vi "O2 main.vi"() -> ()   [LabVIEW 2020, in "O2 Dichtheitstest.lvlib"]
uses:
  O2 Dichtheitstest.lvlib
  O2 Settings.ctl
  Visualisierungs Elemente/Auswahlfeld.ctl
  Aktion O2 Test.ctl
  Aktion FGV O2 Leak.ctl
  Seiten/FT-IR/FGV FT-IR Gasliste Aktionen.ctl
  Seiten/CalGas Aufschaltung/FGV CalGas Aktionen.ctl
  Sprachverwaltung/FGV Aktion Tabelle zerlegen.ctl
  Messdaten/Aktionen FGV Messdaten.ctl
  Funktionstasten/Funktionstasten-Aktion.ctl
  Funktionstasten/Zustaende.ctl
  Seiten/FT-IR/FGV FT-IR Parameter.vi
  Allgemein/allgemeine Sub-VIs.lvlib
  Seiten/FT-IR/FT-IR.lvlib
  Funktionstasten/Funktionstasten.lvlib
  Seiten/CalGas Aufschaltung/CalGas Aufschaltung.lvlib
  Messdaten/Messdaten.lvlib
  Seiten/Grafik/Grafik.lvlib
  Linearisierung V2/Protokoll/Protokoll.lvlib
  Sprachverwaltung/Sprachverwaltung.lvlib
panel:
  out "Result: O2 2":sgl caption="Ergebnis: O2" format="%#.3f"
  out "Messgasdruck":sgl format="%.3f"
  out "Bestanden MGD":bool caption="Boolesch"
  out "Bestanden O2":bool caption="Boolesch"
  out "Graph":waveform(dbl)(graph) caption="Graph1"
  out "Index":i32
  out "Result: Meassuring gas pressure":sgl caption="Ergebnis: Messgasdruck" format="%#.1f"
  out "O2":sgl format="%.3f"
  out "Zeit":sgl
  in  "Textname:":string
  in  "Pfad:":path=path "D:/IAG_Data/Log"
  in  "Speichern":bool
  out "Result: O2":sgl caption="Ergebnis: O2" format="%#.3f"
  in  "Abbrechen":bool
  in  "Test Start":bool
  out "Status":string
  in  "O2 Settings":T1 {"Grenzwert: Messgasdruck 2" format="%#.1f"; "Grenzwert: Messgasdruck" format="%#.1f"; "Grenzwert: O2" format="%#.3f"; "Datenerfassungszeit:" format="%#.1f"; "Nullgas Aufschaltzeit:" format="%#.1f"; "Aufschaltpunkt" items=["Filterblock", "Analysator direkt", "PNS", "Entnahme", "Gasdivider"]; "Kalibriergas" items=["Stickstoff"]}
  # "kPa"
  # "sec"
  # "%"
  # "%"
  # "kPa"
  # "Protokoll"
  # "Ergebnis"
  # "Test - Sequenz"
  # "sec"
  # "%"
  # "-"
  # "kPa"
  # "kPa"
  # "Einstellungen"
  # "O2 Dichtheitstest"
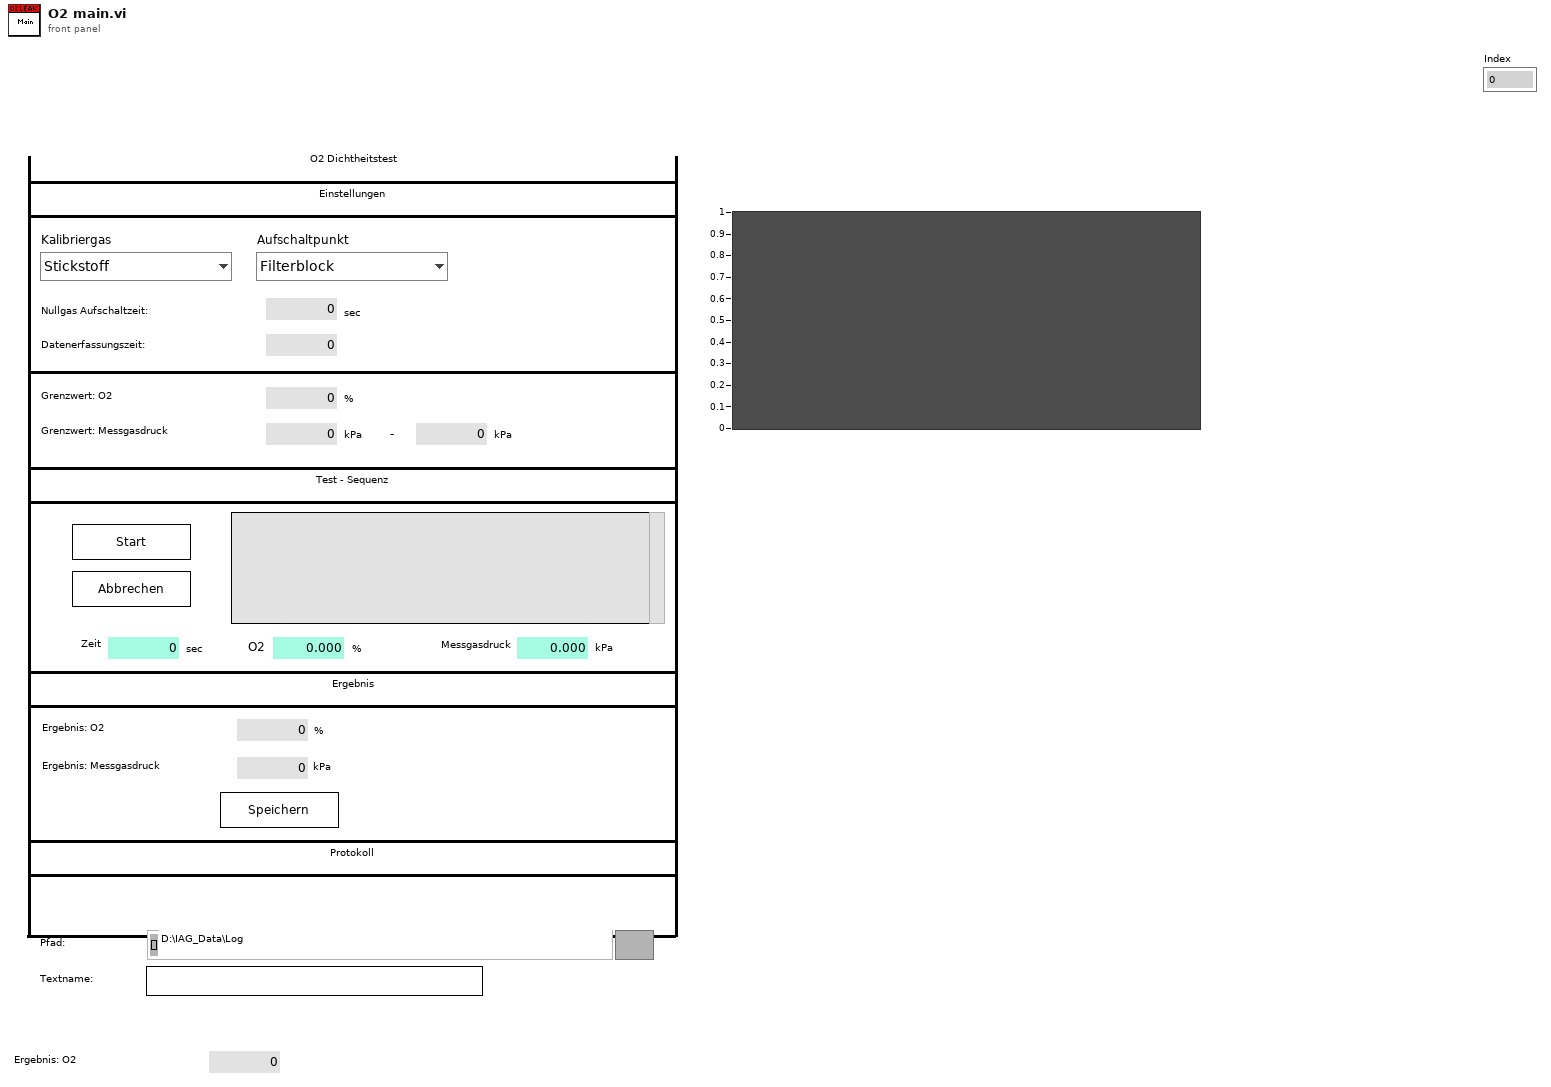
[diagram p1: front panel]
types:
  T1 = typedef "O2 Dichtheitstest.lvlib/O2 Settings.ctl" = cluster{"Kalibriergas":T2, "Aufschaltpunkt":T2, "Nullgas Aufschaltzeit:":sgl, "Datenerfassungszeit:":sgl, "Grenzwert: O2":sgl, "Grenzwert: Messgasdruck":sgl, "Grenzwert: Messgasdruck 2":sgl}
  T2 = typedef "Auswahlfeld.ctl" = u16
  T3 = typedef "O2 Dichtheitstest.lvlib/Aktion O2 Test.ctl" = enum16{"lesen", "ini", "0-Gas", "Auswerten", "Fertig"}
  T4 = typedef "Sprachverwaltung.lvlib/FGV Aktion Tabelle zerlegen.ctl" = enum16{"laden", "vereinzeln", "speichern"}
  T5 = typedef "CalGas Aufschaltung.lvlib/FGV CalGas Aktionen.ctl" = enum16{"lesen", "Analysator Auswahl", "Def.CalGas", "Aufschaltung CalGas", "laden", "speichern", "KAL extrahieren"}
  T6 = enum8{"Enabled", "Disabled", "Disabled and Grayed Out"}
  T7 = typedef "FT-IR.lvlib/FGV FT-IR Gasliste Aktionen.ctl" = enum16{"lesen", "Gasliste FT-IR", "Gasliste ausgelesen", "laden", "speichern", "löschen"}
  T8 = typedef "O2 Dichtheitstest.lvlib/Aktion FGV O2 Leak.ctl" = enum16{"lesen", "O2 settings", "Pfad", "Protokoll", "laden", "speichern"}
  T9 = typedef "String - Ausgabefeld.ctl" = string
  T10 = typedef "CalGas Aufschaltung.lvlib/Definition CalGas Anzeige.ctl" = cluster{"Namen":T11, "Werte":T13, "Werte 2":T13, "Einheit":T15, "Messbereiche":T16}
  T11 = typedef "CalGas Aufschaltung.lvlib/CalGas-Namen.ctl" = cluster{"Name":T12, "Name 2":T12, "Name 3":T12, "Name 4":T12, "Name 5":T12, "Name 6":T12, "Name 7":T12, "Name 8":T12, "Name 9":T12, "Name 10":T12, "Name 11":T12, "Name 12":T12}
  T12 = typedef "String - Eingabefeld.ctl" = string
  T13 = typedef "CalGas Aufschaltung.lvlib/CalGas-Werte.ctl" = cluster{"Konzentration 1":T14, "Konzentration 2":T14, "Konzentration 3":T14, "Konzentration 4":T14, "Konzentration 5":T14, "Konzentration 6":T14, "Konzentration 7":T14, "Konzentration 8":T14, "Konzentration 9":T14, "Konzentration 10":T14, "Konzentration 11":T14, "Konzentration 12":T14}
  T14 = typedef "Zahlen-Eingabefeld.ctl" = sgl
  T15 = typedef "CalGas Aufschaltung.lvlib/CalGas-Einheit.ctl" = cluster{"Einheit 1":T2, "Einheit 2":T2, "Einheit 3":T2, "Einheit 4":T2, "Einheit 5":T2, "Einheit 6":T2, "Einheit 7":T2, "Einheit 8":T2, "Einheit 9":T2, "Einheit 10":T2, "Einheit 11":T2, "Einheit 12":T2}
  T16 = typedef "CalGas Aufschaltung.lvlib/CalGas-Messbereiche.ctl" = cluster{"Messbereich 1":T2, "Messbereich 2":T2, "Messbereich 3":T2, "Messbereich 4":T2, "Messbereich 5":T2, "Messbereich 6":T2, "Messbereich 7":T2, "Messbereich 8":T2, "Messbereich 9":T2, "Messbereich 10":T2, "Messbereich 11":T2, "Messbereich 12":T2}
  T17 = typedef "Messdaten.lvlib/Aktionen FGV Messdaten.ctl" = enum16{"lesen", "schreiben", "löschen", "Mittelwerte", "Komponente"}
  T18 = typedef "Funktionstasten.lvlib/Zustaende.ctl" = enum16{"Standby", "Pause", "Eco", "Messen", "Kalibrieren", "Spülen Filter", "Spülen Leitung", "Umgebungsluft", "0-Gas", "Cal-Gas", "CG zu PNS", "-------------", "Init 1", "Init 2", "Init 3", "Init 4", "Messen vorbereiten", "Messen durchführen", "Exit"}
  T19 = typedef "Funktionstasten.lvlib/Funktionstasten-Aktion.ctl" = enum16{"Initialisieren", "Zustand setzen", "Taste gedrückt", "Fehler speichern", "Lesen", "Manuell", "Remote", "Bitparallel", "Samplepoint", "Zeit Prüfen", "reset Umschalten"}
  T20 = typedef "O2 Dichtheitstest.lvlib/Protokoll LeakTest.ctl" = cluster{"O2":sgl, "Messgasdruck":sgl, "Startzeit":timestamp, "Endzeit":timestamp, "Bestanden?":bool}
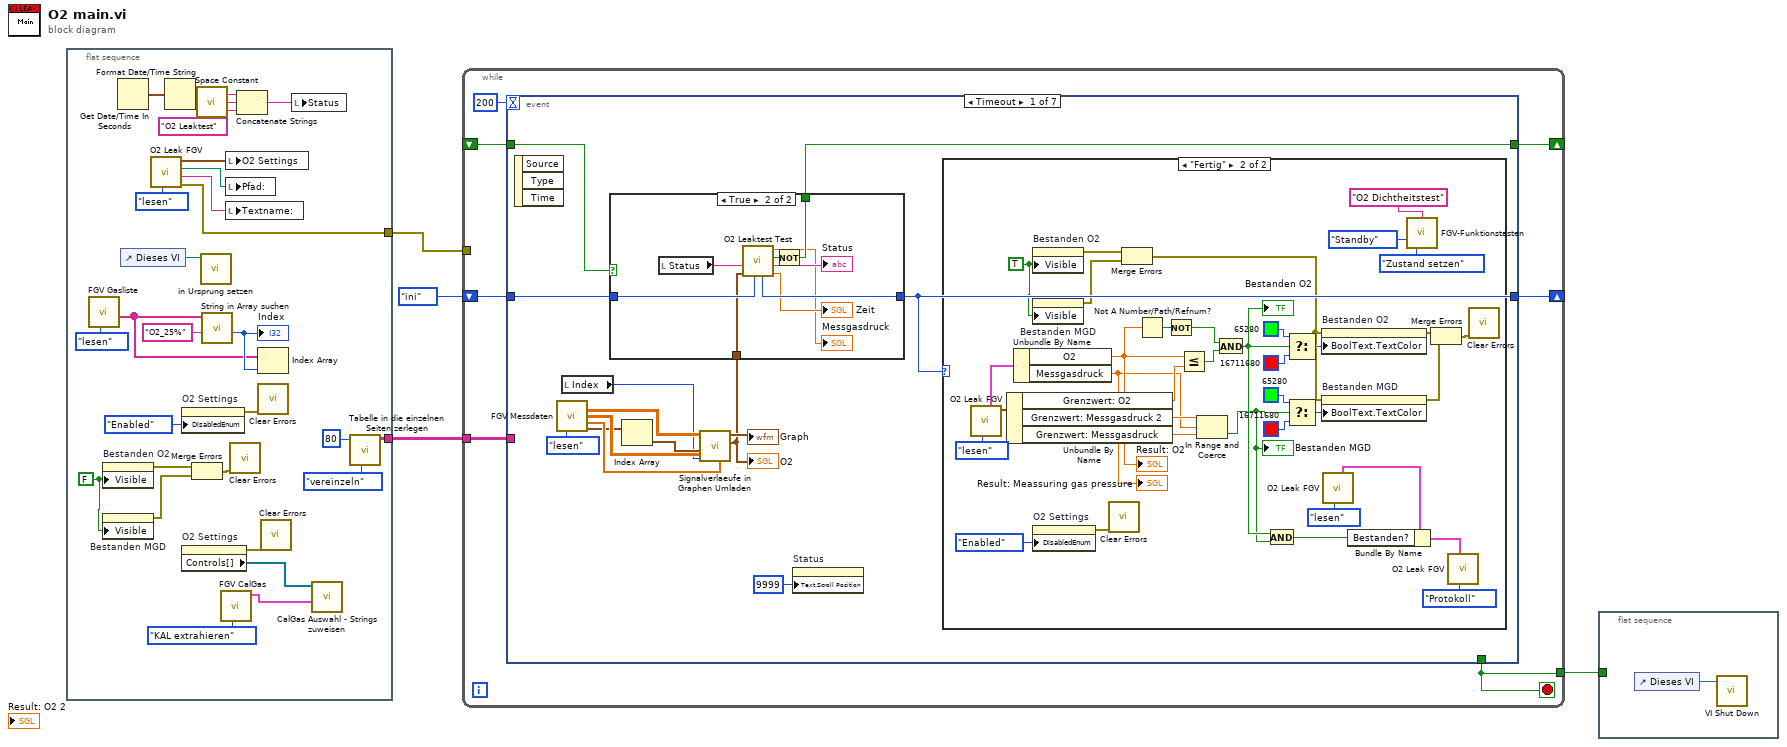
[diagram p0: block diagram]
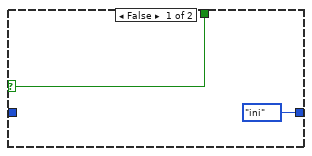
[diagram p3: hidden frame]
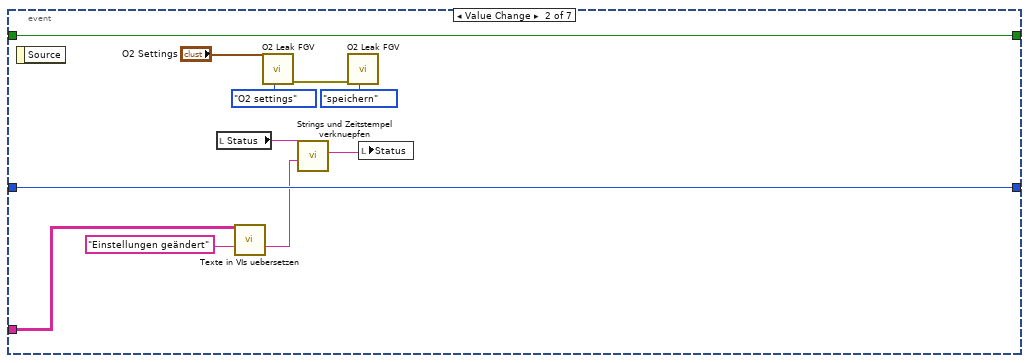
[diagram p4: hidden frame]
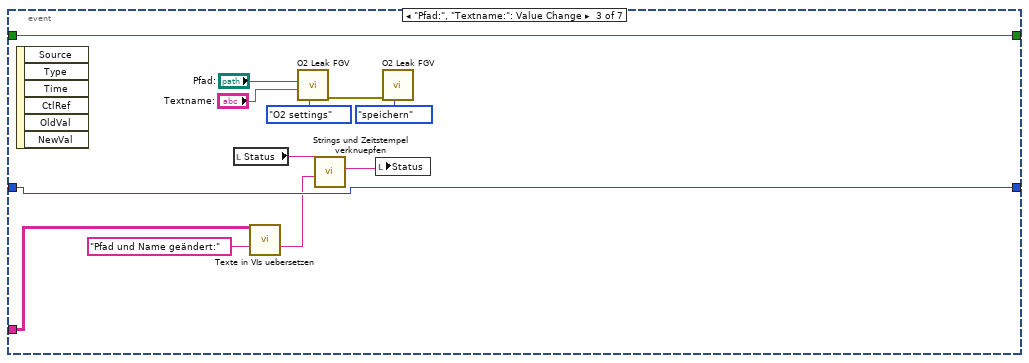
[diagram p5: hidden frame]
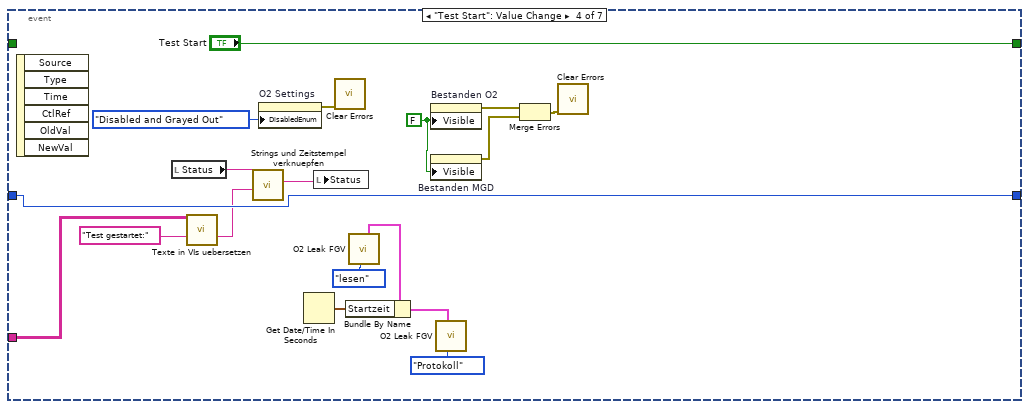
[diagram p6: hidden frame]
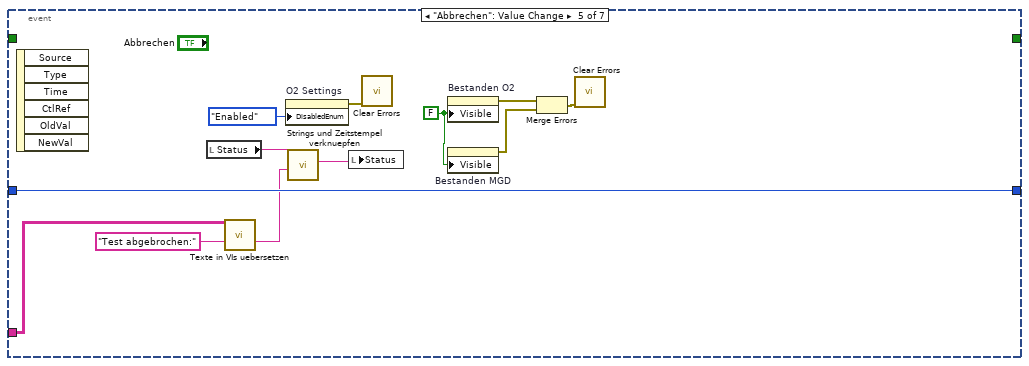
[diagram p7: hidden frame]
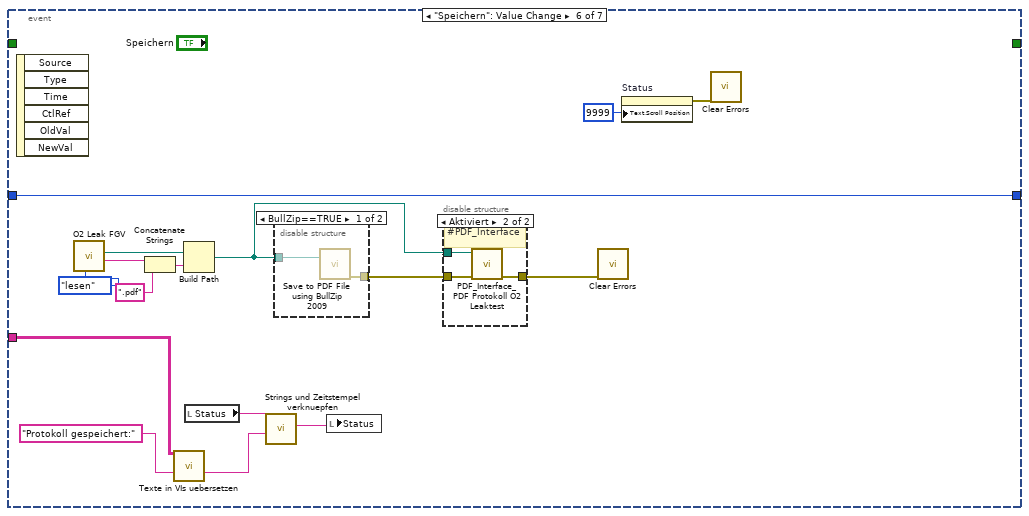
[diagram p8: hidden frame]
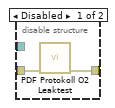
[diagram p9: hidden frame]
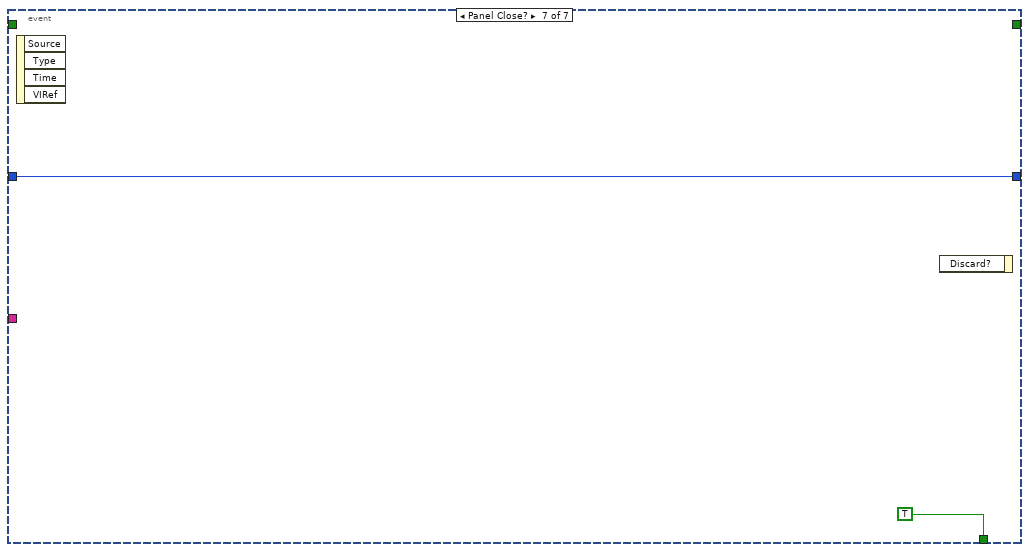
[diagram p11: hidden frame]
diagram:
  n1 = flat-sequence {
    tunnel: [w18] -> w2
    tunnel: [w5] -> w1
    frame #0 {
      w15 = FALSE ("Sichtbar")
      n2 = call "FGV Gasliste.vi"("Aktionen"=FGV_FT-IR_Gasliste_Aktionen."lesen") -> ("Aktuelle Gasliste gesamt"=w22:T9[])  [unwired: 8 in, 2 out]
      n3 = property on="Bestanden O2" class="Bool. (strikt)"("Visible"=w15) -> (error out=w13:errorcluster)  [unwired: 2 in, 1 out]
      n4 = property on="Bestanden MGD" class="Bool. (strikt)"("Visible"=w15) -> (error out=w14:errorcluster)  [unwired: 2 in, 1 out]
      n5 = Get Date/Time In Seconds() -> (seconds since 1Jan1904=w31:timestamp)
      n6 = control-ref of="Dieses VI"() -> (w26:refnum<vi>)
      n7 = call "O2 Leak FGV.vi"("Aktion"=Aktion_FGV_O2_Leak."lesen") -> ("error out"=w18:errorcluster, "Textname:"=w19:string, "Pfad:"=w20:path, "O2 Settings"=w21:T1)  [unwired: 6 in, 1 out]
      n8 = Format Date/Time String(seconds (now)=w31) -> (date/time string=w30:string)  [unwired: 2 in]
      n9 = property on="O2 Settings" class="Cluster (strikt)"("DisabledEnum"=T6."Enabled" ("Deaktiviert")) -> (error out=w16:errorcluster)  [unwired: 2 in, 1 out]
      n10 = property on="O2 Settings" class="Cluster (strikt)"() -> (error out=w8:errorcluster, "Controls[]"=w9:refnum<vi>[])  [unwired: 2 in, 1 out]
      n11 = Merge Errors(w13, w14) -> (w12:errorcluster)
      n12 = call <vilib>:"Space Constant.vi"() -> ("String"=w29:string)
      n13 = call "in Ursprung setzen.vi"("VI Referenz"=w26) -> ()  [unwired: 10 in, 1 out]
      n14 = call "String in Array suchen.vi"("Nach String/Zeichen suchen (-)"="O2_25%", "String-Array"=w22) -> ("Index"=w25:i32)  [unwired: 7 in, 2 out]
      "Index" <- w25
      n15 = call "FGV CalGas.vi"("Aktionen"=FGV_CalGas_Aktionen."KAL extrahieren") -> ("Def.CalGas"=w10:T10)  [unwired: 6 in, 4 out]
      n16 = local write "O2 Settings"(w21) -> ()
      n17 = local write "Pfad:"(w20) -> ()
      n18 = local write "Textname:"(w19) -> ()
      n19 = call <vilib>:"Clear Errors.vi"("error in (no error)"=w12) -> ()  [unwired: 5 in, 2 out]
      n20 = Concatenate Strings(w30, w29, "O2 Leaktest" ("String")) -> (w27:string)
      n21 = Index Array(array=w22, index=w25) -> ()  [unwired: 1 out]
      n22 = call <vilib>:"Clear Errors.vi"("error in (no error)"=w16) -> ()  [unwired: 5 in, 2 out]
      n23 = call <vilib>:"Clear Errors.vi"("error in (no error)"=w8) -> ()  [unwired: 5 in, 2 out]
      n24 = local write "Status"(w27) -> ()
      n25 = call "CalGas Auswahl - Strings zuweisen.vi"("Def.CalGas"=w10, "Aufschaltung CalGas"=w9) -> ()  [unwired: 9 in, 1 out]
      n26 = call "Tabelle in die einzelnen Seiten zerlegen.vi"("Aktion"=FGV_Aktion_Tabelle_zerlegen."vereinzeln", "Index (Seite)"=80) -> ("Sprachliste"=w5:string[][])  [unwired: 7 in, 2 out]
    }
  }
  n27 = while {
    tunnel: [w39] -> w4
    shift-right: [w38] -> _
    shift-left: _ -> [w37]
    shift-right: [w36] -> _
    shift-left: Aktion_O2_Test."ini" ("Aktion") -> [w35]
    tunnel: w2 -> [_]
    tunnel: w1 -> [w33]
    stop <- w39 stop-if-true
    n28 = event shown="[0] Timeout" {
      selector: _ -> [_ _ _ _ _ _ _]
      dyn-events: _ -> [_ _ _ _ _ _ _]
      timeout: 200 -> [_ _ _ _ _ _ _]
      tunnel: [_ _ _ _ _ _ TRUE] -> w39
      tunnel: [w51 w105 w118 "Test Start" _ _ _] -> w38
      tunnel: w37 -> [w53 w105 w118 _ _ _ _]
      tunnel: [w50 w104 w115 w136 w149 w167 w177] -> w36
      tunnel: w35 -> [w52 w104 w115 w136 w149 w167 w177]
      tunnel: w33 -> [_ w101 w112 w124 w142 w160 _]
      event Timeout {
        n29 = event-data() -> ()  [unwired: 1 in, 3 out]
        n30 = call "FGV Messdaten.vi"("Aktionen"=Aktionen_FGV_Messdaten."lesen") -> ("Messdaten"=w46:sgl[][], "Mittelwertdaten"=w48:sgl[][], "Deviation"=w49:sgl[], "Zeitstempeln"=w44:timestamp[])  [unwired: 6 in, 5 out]
        n31 = local read "Index"() -> (w42:i32)
        n32 = Index Array(array=w44) -> (element=w47:timestamp)  [unwired: 1 in]
        n33 = call "Signalverlaeufe in Graphen Umladen.vi"("Deviation"=w49, "Mittelwertdaten"=w48, "Gas-Auswahl"=w42, "t0"=w47, "Werte"=w46) -> ("Mittelwert"=w41:waveform(dbl), "Waveform"=→"Graph":waveform(dbl))  [unwired: 2 in, 3 out]
        "O2" <- w41
        n34 = case shown="True" w53 {
          selector: w53 -> [w90 _]
          tunnel: [Aktion_O2_Test."ini" ("Aktion") w100] -> w50
          tunnel: w52 -> [_ w99]
          tunnel: [w90 w95] -> w51
          tunnel: w41 -> [_ w93]
          frame False {
          }
          frame True {
            n35 = local read "Status"() -> (w98:string)
            n36 = call "O2 Leaktest Test.vi"("Aktion"=w99, "O2"=w93, "Status"=w98) -> ("countdown"=→"Zeit":dbl, "Status"=→"Status":string, "Fertig?"=w96:bool, "Messgasdruck"=→"Messgasdruck":sgl, "Aktion"=w100:T3)  [unwired: 4 in]
            n37 = Not(x=w96) -> (.not. x?=w95:bool)
          }
        }
        n38 = property on="Status" class="Str"("Text.Scroll Position"=u32 9999 ("Text.Anzeigeposition")) -> ()  [unwired: 2 in, 2 out]
        n39 = case shown="\"Fertig\"" w50 {
          frame "lesen", Default {
          }
          frame "Fertig" {
            w72 = TRUE ("Sichtbar")
            n40 = call "O2 Leak FGV.vi"("Aktion"=Aktion_FGV_O2_Leak."lesen") -> ("O2 Settings"=w88:T1, "Protokoll"=w87:T20)  [unwired: 6 in, 3 out]
            n41 = Unbundle By Name(w88) -> ("Grenzwert: O2"=w86:sgl, "Grenzwert: Messgasdruck 2"=w56:sgl, "Grenzwert: Messgasdruck"=w57:sgl)
            n42 = Unbundle By Name(w87) -> ("O2"=w62:sgl, "Messgasdruck"=w55:sgl)
            "Result: O2" <- w62
            "Result: Meassuring gas pressure" <- w55
            n43 = property on="Bestanden O2" class="Bool. (strikt)"("Visible"=w72) -> (error out=w70:errorcluster)  [unwired: 2 in, 1 out]
            n44 = property on="Bestanden MGD" class="Bool. (strikt)"("Visible"=w72) -> (error out=w71:errorcluster)  [unwired: 2 in, 1 out]
            n45 = property on="O2 Settings" class="Cluster (strikt)"("DisabledEnum"=T6."Enabled" ("Deaktiviert")) -> (error out=w67:errorcluster)  [unwired: 2 in, 1 out]
            n46 = call <vilib>:"Clear Errors.vi"("error in (no error)"=w67) -> ()  [unwired: 5 in, 2 out]
            n47 = Merge Errors(w70, w71) -> (w63:errorcluster)
            n48 = Not A Number/Path/Refnum?(number/path/refnum=w62) -> (NaN/Path/Refnum?=w61:bool)
            n49 = Not(x=w61) -> (.not. x?=w59:bool)
            n50 = Less Or Equal?(x=w62, y=w86) -> (x <= y?=w60:bool)
            n51 = In Range and Coerce(upper limit=w56, x=w55, lower limit=w57) -> (In Range?=w54:bool)  [unwired: 1 out]
            "Bestanden MGD" <- w54
            n52 = And(x=w59, y=w60) -> (x .and. y?=w58:bool)
            "Bestanden O2" <- w58
            n53 = And(x=w58, y=w54) -> (x .and. y?=w75:bool)
            n54 = Select(t=u32 65280, s=w58, f=u32 16711680) -> (s? t:f=w69:u32)
            n55 = Select(t=u32 65280, s=w54, f=u32 16711680) -> (s? t:f=w81:u32)
            n56 = property on="Bestanden O2" class="Bool. (strikt)"(error in=w63, "BoolText.TextColor"=w69) -> (error out=w80:errorcluster)  [unwired: 1 in, 1 out]
            n57 = property on="Bestanden MGD" class="Bool. (strikt)"(error in=w63, "BoolText.TextColor"=w81) -> (error out=w79:errorcluster)  [unwired: 1 in, 1 out]
            n58 = call "O2 Leak FGV.vi"("Aktion"=Aktion_FGV_O2_Leak."lesen") -> ("Protokoll"=w76:T20)  [unwired: 6 in, 4 out]
            n59 = Bundle By Name(cluster=w76, "Bestanden?"=w75) -> (w73:T20)
            n60 = call "FGV-Funktionstasten.vi"("Herkunft"="O2 Dichtheitstest", "Zustand"=Zustaende."Standby", "Aktion"=Funktionstasten-Aktion."Zustand setzen") -> ()  [unwired: 5 in, 8 out]
            n61 = Merge Errors(w80, w79) -> (w78:errorcluster)
            n62 = call "O2 Leak FGV.vi"("Aktion"=Aktion_FGV_O2_Leak."Protokoll", "Protokoll"=w73) -> ()  [unwired: 5 in, 5 out]
            n63 = call <vilib>:"Clear Errors.vi"("error in (no error)"=w78) -> ()  [unwired: 5 in, 2 out]
          }
        }
      }
      event Value Change {
        n64 = event-data() -> ()  [unwired: 1 in, 1 out]
        n65 = local read "Status"() -> (w106:string)
        n66 = call "Texte in VIs uebersetzen.vi"("Sprachliste"=w101, "String zum Übersetzen"="Einstellungen geändert" ("String 1 hinzufügen")) -> ("String zum Übersetzen"=w102:string)  [unwired: 9 in, 4 out]
        n67 = call "O2 Leak FGV.vi"("Aktion"=Aktion_FGV_O2_Leak."O2 settings", "O2 Settings"="O2 Settings") -> ("error out"=w108:errorcluster)  [unwired: 5 in, 4 out]
        n68 = call "Strings und Zeitstempel verknuepfen.vi"("String 1 hinzufügen"=w102, "Eingagns String"=w106) -> ("Verknüpfter String"=w107:string)  [unwired: 9 in]
        n69 = call "O2 Leak FGV.vi"("Aktion"=Aktion_FGV_O2_Leak."speichern", "error in (no error)"=w108) -> ()  [unwired: 5 in, 5 out]
        n70 = local write "Status"(w107) -> ()
      }
      event "Pfad:", "Textname:": Value Change {
        n71 = event-data() -> ()  [unwired: 1 in, 6 out]
        n72 = local read "Status"() -> (w116:string)
        n73 = call "Texte in VIs uebersetzen.vi"("Sprachliste"=w112, "String zum Übersetzen"="Pfad und Name geändert:" ("String 1 hinzufügen")) -> ("String zum Übersetzen"=w113:string)  [unwired: 9 in, 4 out]
        n74 = call "O2 Leak FGV.vi"("Aktion"=Aktion_FGV_O2_Leak."O2 settings", "Textname:"="Textname:", "Pfad:"="Pfad:") -> ("error out"=w121:errorcluster)  [unwired: 4 in, 4 out]
        n75 = call "Strings und Zeitstempel verknuepfen.vi"("String 1 hinzufügen"=w113, "Eingagns String"=w116) -> ("Verknüpfter String"=w117:string)  [unwired: 9 in]
        n76 = local write "Status"(w117) -> ()
        n77 = call "O2 Leak FGV.vi"("Aktion"=Aktion_FGV_O2_Leak."speichern", "error in (no error)"=w121) -> ()  [unwired: 5 in, 5 out]
      }
      event "Test Start": Value Change {
        w135 = FALSE ("Sichtbar")
        n78 = event-data() -> ()  [unwired: 1 in, 6 out]
        n79 = local read "Status"() -> (w137:string)
        n80 = call "Texte in VIs uebersetzen.vi"("Sprachliste"=w124, "String zum Übersetzen"="Test gestartet:" ("String 1 hinzufügen")) -> ("String zum Übersetzen"=w125:string)  [unwired: 9 in, 4 out]
        n81 = call "Strings und Zeitstempel verknuepfen.vi"("String 1 hinzufügen"=w125, "Eingagns String"=w137) -> ("Verknüpfter String"=w138:string)  [unwired: 9 in]
        n82 = property on="O2 Settings" class="Cluster (strikt)"("DisabledEnum"=T6."Disabled and Grayed Out" ("Deaktiviert")) -> (error out=w139:errorcluster)  [unwired: 2 in, 1 out]
        n83 = Get Date/Time In Seconds() -> (seconds since 1Jan1904=w127:timestamp)
        n84 = local write "Status"(w138) -> ()
        n85 = call <vilib>:"Clear Errors.vi"("error in (no error)"=w139) -> ()  [unwired: 5 in, 2 out]
        n86 = call "O2 Leak FGV.vi"("Aktion"=Aktion_FGV_O2_Leak."lesen") -> ("Protokoll"=w129:T20)  [unwired: 6 in, 4 out]
        n87 = Bundle By Name(cluster=w129, "Startzeit"=w127) -> (w128:T20)
        n88 = property on="Bestanden O2" class="Bool. (strikt)"("Visible"=w135) -> (error out=w133:errorcluster)  [unwired: 2 in, 1 out]
        n89 = property on="Bestanden MGD" class="Bool. (strikt)"("Visible"=w135) -> (error out=w134:errorcluster)  [unwired: 2 in, 1 out]
        n90 = call "O2 Leak FGV.vi"("Aktion"=Aktion_FGV_O2_Leak."Protokoll", "Protokoll"=w128) -> ()  [unwired: 5 in, 5 out]
        n91 = Merge Errors(w133, w134) -> (w132:errorcluster)
        n92 = call <vilib>:"Clear Errors.vi"("error in (no error)"=w132) -> ()  [unwired: 5 in, 2 out]
      }
      event "Abbrechen": Value Change {
        w148 = FALSE ("Sichtbar")
        n93 = event-data() -> ()  [unwired: 1 in, 6 out]
        n94 = local read "Status"() -> (w150:string)
        n95 = call "Texte in VIs uebersetzen.vi"("Sprachliste"=w142, "String zum Übersetzen"="Test abgebrochen:" ("String 1 hinzufügen")) -> ("String zum Übersetzen"=w143:string)  [unwired: 9 in, 4 out]
        n96 = property on="O2 Settings" class="Cluster (strikt)"("DisabledEnum"=T6."Enabled" ("Deaktiviert")) -> (error out=w152:errorcluster)  [unwired: 2 in, 1 out]
        n97 = call "Strings und Zeitstempel verknuepfen.vi"("String 1 hinzufügen"=w143, "Eingagns String"=w150) -> ("Verknüpfter String"=w151:string)  [unwired: 9 in]
        n98 = local write "Status"(w151) -> ()
        n99 = call <vilib>:"Clear Errors.vi"("error in (no error)"=w152) -> ()  [unwired: 5 in, 2 out]
        n100 = property on="Bestanden O2" class="Bool. (strikt)"("Visible"=w148) -> (error out=w146:errorcluster)  [unwired: 2 in, 1 out]
        n101 = property on="Bestanden MGD" class="Bool. (strikt)"("Visible"=w148) -> (error out=w147:errorcluster)  [unwired: 2 in, 1 out]
        n102 = Merge Errors(w146, w147) -> (w145:errorcluster)
        n103 = call <vilib>:"Clear Errors.vi"("error in (no error)"=w145) -> ()  [unwired: 5 in, 2 out]
      }
      event "Speichern": Value Change {
        n104 = event-data() -> ()  [unwired: 1 in, 6 out]
        n105 = call "O2 Leak FGV.vi"("Aktion"=Aktion_FGV_O2_Leak."lesen") -> ("Textname:"=w158:string, "Pfad:"=w159:path)  [unwired: 6 in, 3 out]
        n106 = Concatenate Strings(w158, ".pdf") -> (w157:string)
        n107 = call "Texte in VIs uebersetzen.vi"("Sprachliste"=w160, "String zum Übersetzen"="Protokoll gespeichert:" ("String 1 hinzufügen")) -> ("String zum Übersetzen"=w161:string)  [unwired: 9 in, 4 out]
        n108 = Build Path(base path=w159, name or relative path=w157) -> (appended path=w154:path)
        n109 = local read "Status"() -> (w168:string)
        n110 = call "Strings und Zeitstempel verknuepfen.vi"("String 1 hinzufügen"=w161, "Eingagns String"=w168) -> ("Verknüpfter String"=w169:string)  [unwired: 9 in]
        n111 = disable-structure shown="BullZip==TRUE" {
          disable-tunnel: [w176 _] -> w163
          disable-tunnel: w154 -> [w175 _]
          frame condition #0 {
            n112 = call "Save to PDF File using BullZip 2009.vi"("Save PDF File Path"=w175) -> ("error out"=w176:errorcluster)  [unwired: 10 in]
          }
          frame condition #1 (active) {
          }
        }
        n113 = local write "Status"(w169) -> ()
        n114 = disable-structure shown="Aktiviert" {
          disable-tunnel: [w171 w173] -> w166
          disable-tunnel: w163 -> [w170 w174]
          disable-tunnel: w154 -> [_ w172]
          frame Disabled {
            n115 = call "PDF Protokoll O2 Leaktest.vi"("error in (no error)"=w170) -> ("error out"=w171:errorcluster)  [unwired: 10 in]
          }
          frame Enabled {
            # "#PDF_Interface"
            n116 = call "PDF_Interface_PDF Protokoll O2 Leaktest.vi"("error in (no error)"=w174, "Save PDF File Path"=w172) -> ("error out"=w173:errorcluster)  [unwired: 9 in]
          }
        }
        n117 = call <vilib>:"Clear Errors.vi"("error in (no error)"=w166) -> ()  [unwired: 5 in, 2 out]
        n118 = property on="Status" class="Str"("Text.Scroll Position"=u32 9999 ("Text.Anzeigeposition")) -> (error out=w164:errorcluster)  [unwired: 2 in, 1 out]
        n119 = call <vilib>:"Clear Errors.vi"("error in (no error)"=w164) -> ()  [unwired: 5 in, 2 out]
      }
      event Panel Close? {
        n120 = event-data() -> ()  [unwired: 1 in, 4 out]
        n121 = event-data() -> ()  [unwired: 2 in, 1 out]
      }
    }
  }
  n122 = flat-sequence {
    tunnel: w4 -> [_]
    frame #0 {
      n123 = control-ref of="Dieses VI"() -> (w179:refnum<vi>)
      n124 = call "VI Shut Down.vi"("VI Referenz"=w179) -> ()  [unwired: 11 in]
    }
  }
